vi "Get Top Target Information.vi"(0 "Vision Info Array":dbl[][](array[numeric])) -> (1 "Center of Mass X":dbl)   [LabVIEW 2011]
panel:
  # "Analysis"
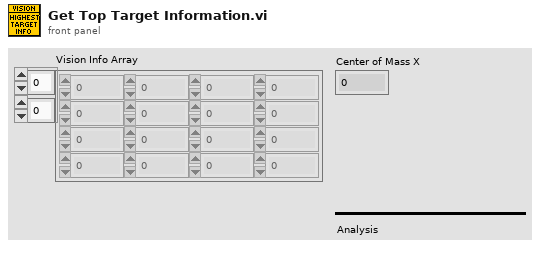
[diagram p1: front panel]
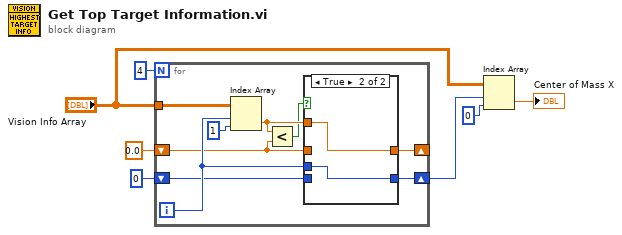
[diagram p0: block diagram]
diagram:
  n1 = for {
    N: 4 -> [_]
    tunnel: "Vision Info Array" -> [w16]
    shift-right: [w11] -> _
    shift-left: 0.0 ("Numeric") -> [w9]
    shift-right: [w13] -> w1
    shift-left: 0 -> [w10]
    i -> [w14]
    n2 = Index Array(array=w16, index (row)=w14, index (col)=1 ("disabled index (col)")) -> (element=w12:dbl)
    n3 = Less?(x=w12, y=w9) -> (x < y?=w8:bool)
    n4 = case shown="True" w8 {
      tunnel: w14 -> [_ w20]
      tunnel: [w18 w20] -> w13
      tunnel: w12 -> [_ w19]
      tunnel: [w17 w19] -> w11
      tunnel: w10 -> [w18 _]
      tunnel: w9 -> [w17 _]
      frame False {
      }
      frame True {
      }
    }
  }
  n5 = Index Array(array="Vision Info Array", index (row)=w1, index (col)=0) -> (element=→"Center of Mass X":dbl)
